vi "Shooter.vi"() -> (2 "Bottom":dbl, 3 "Top":dbl)   [LabVIEW 2019]
uses:
  <vilib>/Rock Robotics/Network Tables/NT Read Number.vi
panel:
  out "Distance":dbl
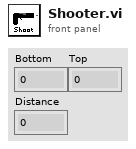
[diagram p1: front panel]
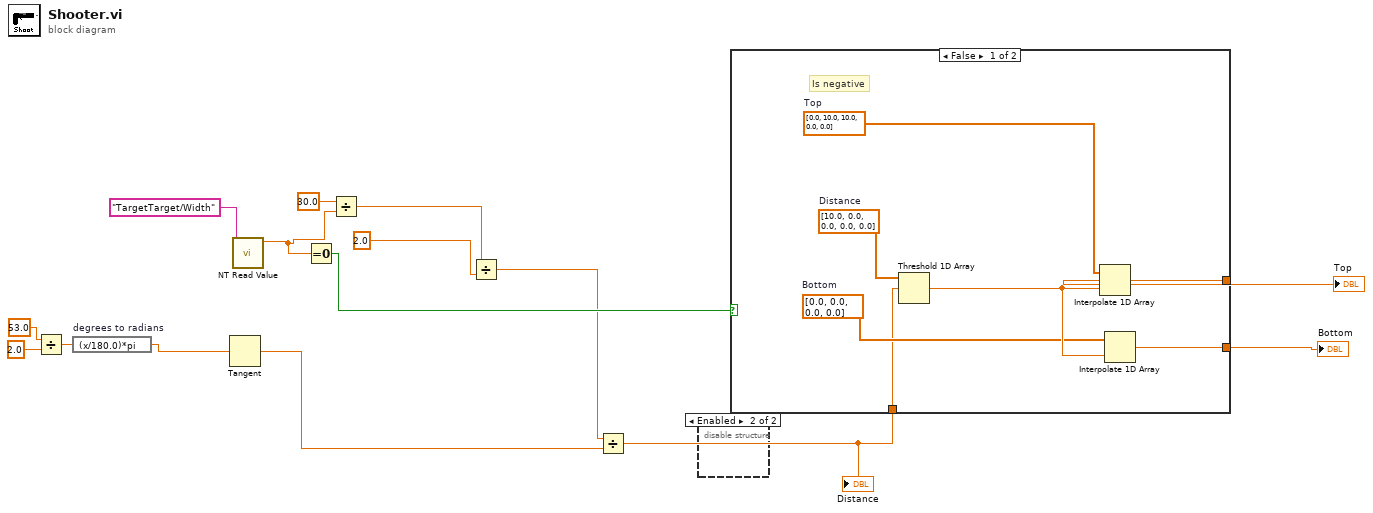
[diagram p0: block diagram]
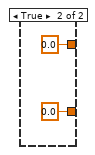
[diagram p3: hidden frame]
diagram:
  n1 = Divide(x=53.0, y=2.0) -> (x/y=w11:dbl)
  n2 = expression code="(x/180.0)*pi" "degrees to radians"(w11) -> (w10:dbl)
  n3 = Tangent(1:w10) -> (0:w4:dbl)
  n4 = call-poly <vilib>:"NT Read Value.vi"("Name"="TargetTarget/Width") -> ("Numeric"=w9:dbl)  [unwired: 9 in, 1 out]
  n5 = Equal To 0?(x=w9) -> (x = 0?=w8:bool)
  n6 = Divide(x=30.0, y=w9) -> (x/y=w5:dbl)
  n7 = Divide(x=w5, y=2.0) -> (x/y=w3:dbl)
  n8 = Divide(x=w3, y=w4) -> (x/y=w2:dbl)
  "Distance" <- w2
  n9 = disable-structure shown="Enabled" {
    frame Disabled {
    }
    frame Enabled {
    }
  }
  n10 = case shown="False" w8 {
    tunnel: [w18 0.0] -> w7
    tunnel: [w17 0.0] -> w1
    tunnel: w2 -> [w16 _]
    frame False {
      w21 = dbl[] [10.0, 0.0, 0.0, 0.0, 0.0]  # Distance
      w19 = dbl[] [0.0, 10.0, 10.0, 0.0, 0.0]  # Top
      w20 = dbl[] [0.0, 0.0, 0.0, 0.0]  # Bottom
      # "Is negative"
      n11 = Threshold 1D Array(2:w16, 3:w21) -> (0:w22:dbl)  [unwired: 1 in]
      n12 = Interpolate 1D Array(1:w22, 2:w19) -> (0:w18:dbl)
      n13 = Interpolate 1D Array(1:w22, 2:w20) -> (0:w17:dbl)
    }
    frame True {
    }
  }
  "Top" <- w7
  "Bottom" <- w1
